vi "Copy.vi"(8 "error in":errorcluster, 10 "Image Dst Reference In":T1, 11 "Image Src Reference In":T1) -> (0 "error out":errorcluster, 3 "Image Dst Reference Out":T1)   [LabVIEW 2024, in "OpenLvVision_Image.lvlib" / "Management.lvlib"]
doc: "Creates an independent duplicate of an image, including its pixel data, dimensions, and metadata. Modifications to the copy do not affect the original."
uses:
  Management.lvlib
  TypeDef/Image.ctl
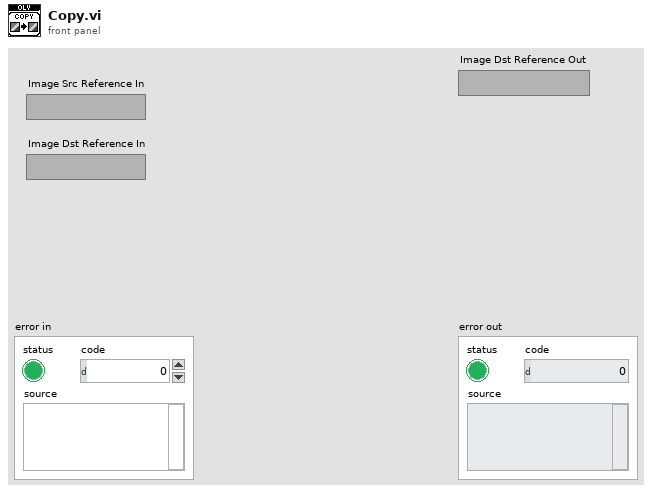
[diagram p1: front panel]
types:
  T1 = typedef "OpenLvVision_Image.lvlib/Management.lvlib/Image.ctl" = refnum<image>
  T2 = typedef "IMAQ Image.ctl" = refnum<image>
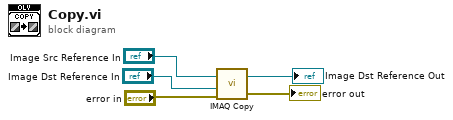
[diagram p0: block diagram]
diagram:
  n1 = call "IMAQ Copy"("error in (no error)"="error in", "Image Dst"="Image Dst Reference In", "Image Src"="Image Src Reference In") -> ("error out"=→"error out":errorcluster, "Image Dst Out"=→"Image Dst Reference Out":T2)  [unwired: 3 in]
